vi "Message Set Module Address.vi"(0 "Port":u16=65535, 1 "Address":string, 2 "Module":string) -> ()   [LabVIEW 2019]
uses:
  e1039-target-controls/PDP/Utility VI's/Message VI's/Message Address Global.vi
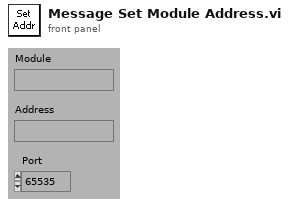
[diagram p1: front panel]
types:
  T1 = cluster{"Module":string, "Address":string, "Port":u16}[]
  T2 = cluster{"Module":string, "Address":string, "Port":u16}
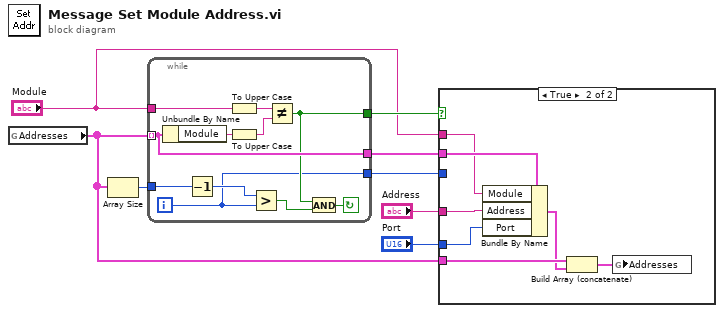
[diagram p0: block diagram]
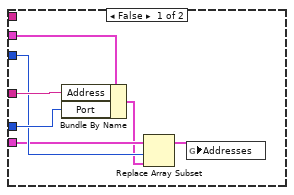
[diagram p2: hidden frame]
diagram:
  n1 = global read "Message Address Global.vi" "Addresses"() -> (w6:T1)
  n2 = Array Size(array=w6) -> (size(s)=w8:i32)
  n3 = while {
    tunnel: [w9] -> w2
    tunnel: [w13] -> w7
    tunnel: [w14] -> w3
    tunnel: w8 -> [w15]
    tunnel: "Module" -> [w18]
    tunnel: w6 -> [w14] mode=indexing
    i -> [w9]
    stop <- w10 continue-if-true
    n4 = Unbundle By Name(w14) -> ("Module"=w19:string)
    n5 = Decrement(x=w15) -> (x-1=w12:i32)
    n6 = To Upper Case(1:w18) -> (0:w17:string)
    n7 = To Upper Case(1:w19) -> (0:w16:string)
    n8 = Greater?(x=w12, y=w9) -> (0:w11:bool)
    n9 = Not Equal?(x=w17, y=w16) -> (x != y?=w13:bool)
    n10 = And(x=w13, y=w11) -> (x .and. y?=w10:bool)
  }
  n11 = case shown="True" w7 {
    tunnel: w6 -> [w22 w29]
    tunnel: "Module" -> [_ w32]
    tunnel: "Port" -> [w24 w30]
    tunnel: w3 -> [w26 w33]
    tunnel: w2 -> [w23 _]
    tunnel: "Address" -> [w25 w31]
    frame False {
      n12 = Bundle By Name(cluster=w26, "Address"=w25, "Port"=w24) -> (w21:T2)
      n13 = Replace Array Subset(array=w22, new element=w21, index=w23) -> (w20:T1)
      n14 = global write "Message Address Global.vi" "Addresses"(w20) -> ()
    }
    frame True {
      n15 = Bundle By Name(cluster=w33, "Module"=w32, "Address"=w31, "Port"=w30) -> (w28:T2)
      n16 = Build Array (concatenate)(w29, w28) -> (w27:T1)
      n17 = global write "Message Address Global.vi" "Addresses"(w27) -> ()
    }
  }
